vi "rs3_MemCopyUINT16_3.vi"(6 "Image format":u16(ring) items=["Y16", "Y8"], 7 "Transpose":bool=TRUE, 8 "error in (no error)":errorcluster, 9 "Height":i32, 10 "Width":i32, 11 "Zimage pointer":u64) -> (0 "error out":errorcluster, 2 "2D Array Output":u16[][](array[numeric]))   [LabVIEW 2023]
doc: "Use this after a Get Frame Data VI to copy the memory pointed to, into an 2D array in LabVIEW.\nThis VI should be used for DEPTH and UNRECT IMAGE data that is 16 or 8 bits."
panel:
  # "RS3_Mem Copy"
  # "(C) 2017 Intel Corp.,  AGJ"
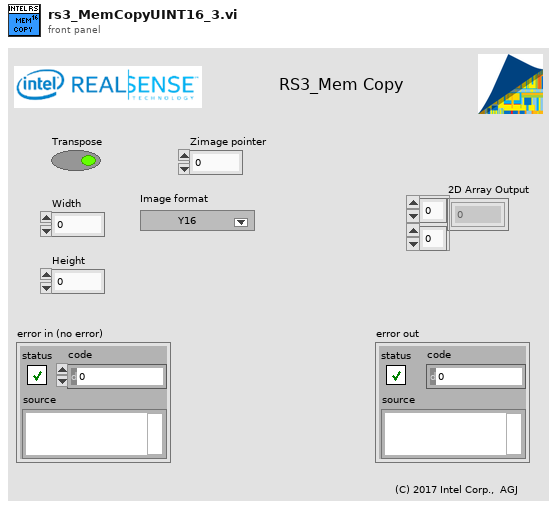
[diagram p1: front panel]
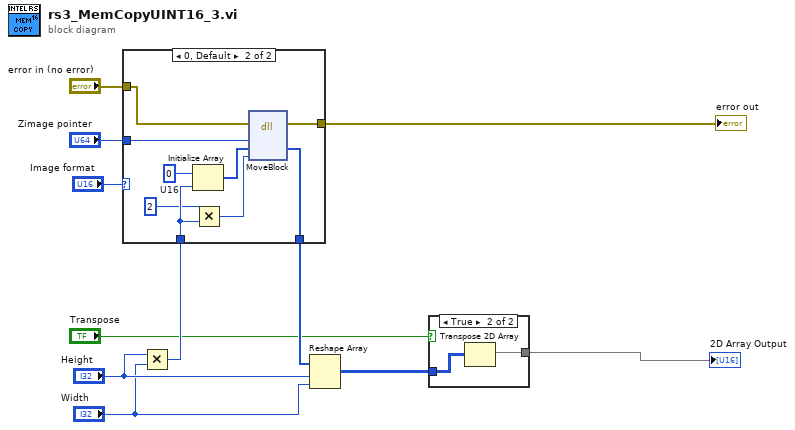
[diagram p0: block diagram]
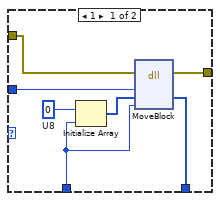
[diagram p3: hidden frame]
diagram:
  n1 = Multiply(x="Height", y="Width") -> (x*y=w5:i32)
  n2 = case shown="0, Default" "Image format" {
    tunnel: [w18 w27] -> w10
    tunnel: [w17 w26] -> w9
    tunnel: "error in (no error)" -> [w16 w25]
    tunnel: w5 -> [w12 w21]
    tunnel: "Zimage pointer" -> [w13 w19]
    frame 1 {
      w15 = u8 0  # U8
      n3 = Initialize Array(w15, w12) -> (w14:u8[])
      n4 = dll-call lib="LabVIEW" fn="MoveBlock"(error in=w16, "Address(Pointer)"=w13, "Destination"=w14, "Size"=w12) -> (error out=w17:errorcluster, "Destination"=w18:u8[])  [unwired: 5 in, 1 out]
    }
    frame 0, Default {
      w24 = u16 0  # U16
      n5 = Initialize Array(w24, w21) -> (w23:u16[])
      n6 = Multiply(x=2 ("factor"), y=w21) -> (x*y=w22:i32)
      n7 = dll-call lib="LabVIEW" fn="MoveBlock"(error in=w25, "Address(Pointer)"=w19, "Destination"=w23, "Size"=w22) -> (error out=w26:errorcluster, "Destination"=w27:u16[])  [unwired: 5 in, 1 out]
    }
  }
  "error out" <- w9
  n8 = Reshape Array(w10, "Height", "Width") -> (w11:u16[][])
  n9 = case shown="True" "Transpose" {
    tunnel: w11 -> [w28 w30]
    tunnel: [w28 w29] -> w2
    frame False {
    }
    frame True {
      n10 = Transpose 2D Array(2D array=w30) -> (transposed array=w29:u16[][])
    }
  }
  "2D Array Output" <- w2
